vi "PTScanner.remove object.vi"(0 "i ref in":refnum<vi>, 2 "index":i32, 5 "error in (no error)":errorcluster) -> (14 "i ref out":refnum<vi>, 19 "error out":errorcluster)   [LabVIEW 2014, in "PTScanner.lvlib"]
uses:
  PTScanner.lvlib
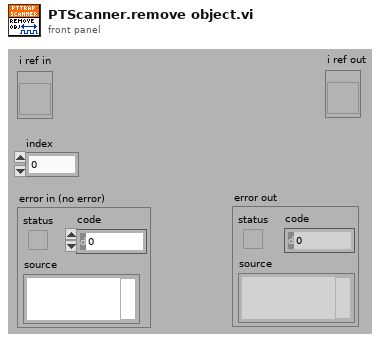
[diagram p1: front panel]
types:
  T1 = typedef "PTScanner.lvlib/PTScanner.i attribute.ctl" = cluster{"Object cmds":T2[], "Steps":cluster{"Finished":bool, "cmd setup":T3[]}[], "curStep":i32, "DIM IDs":cluster{"AllFinished":i32, "Finished":i32, "curStep":i32, "nofSteps":i32, "NomValues":i32[], "1D-Min":i32, "1D-Max":i32, "Dimensions":i32, "MaxDimensions":i32, "ScanedDeviceNames":i32[]}, "All Finished":bool, "DIMs in use":string[], "Running":bool, "Scan Delay":u32, "loop":bool, "Paused":bool, "Formed":bool}
  T2 = typedef "PTScanner.lvlib/PTScanner.obj parameters.ctl" = cluster{"object":string, "DIM address":string, "method":string, "data descriptor":string, "method parameters":cluster{"Name":string, "Descr":string, "Value":string, "Value?":bool}[], "Call Mode":enum16{"Simple DIM", "Synchronous"}, "actValue":dbl, "Centroid":dbl, "Minus Delta":dbl, "Plus Delta":dbl, "increment":dbl, "DIM Status":cluster{"no link":bool, "quality":i32, "Time Stamp":timestamp}, "range":dbl, "DIMChannelIndex":i32}
  T3 = typedef "PTScanner.lvlib/PTScanner.step obj parameters.ctl" = cluster{"obj index":i32, "nomValue":dbl, "fulfilled":bool}
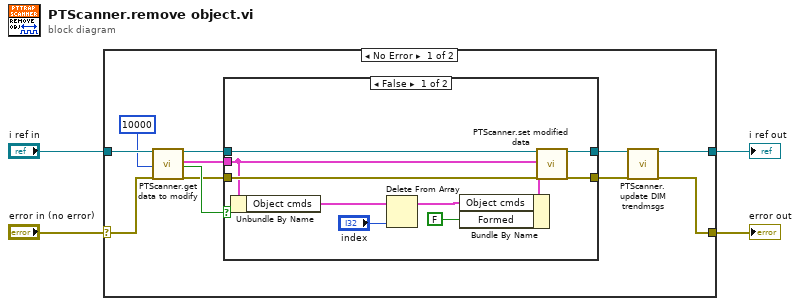
[diagram p0: block diagram]
diagram:
  n1 = case shown="No Error" "error in (no error)" {
    selector: "error in (no error)" -> [w10 w28]
    tunnel: "i ref in" -> [w11 w29]
    tunnel: [w7 w29] -> w2
    tunnel: [w5 w28] -> w1
    frame No Error {
      n2 = call "PTScanner.get data to modify.vi"("i ref in"=w11, "ms timeout (10000)"=10000, "error in (no error)"=w10) -> ("i ref out"=w14:refnum<vi>, "i attribute"=w12:T1, "timed out"=w15:bool, "error out"=w13:errorcluster)  [unwired: 13 in]
      n3 = case shown="False" w15 {
        tunnel: w14 -> [w25 w26]
        tunnel: w13 -> [w24 w27]
        tunnel: w12 -> [w23 _]
        tunnel: [w17 w27] -> w6
        tunnel: [w18 w26] -> w8
        frame False {
          n4 = Unbundle By Name(w23) -> ("Object cmds"=w21:T2[])
          n5 = Delete From Array(array=w21, index="index") -> (array with subset deleted=w20:T2[])  [unwired: 1 in, 1 out]
          n6 = Bundle By Name(cluster=w23, "Object cmds"=w20, "Formed"=FALSE) -> (w22:T1)
          n7 = call "PTScanner.set modified data.vi"("i ref in"=w25, "CLASS.i attribute"=w22, "error in (no error)"=w24) -> ("i ref out"=w18:refnum<vi>, "error out"=w17:errorcluster)  [unwired: 15 in]
        }
        frame True {
        }
      }
      n8 = call "PTScanner.update DIM trendmsgs.vi"("i ref in"=w8, "error in"=w6) -> ("i ref out"=w7:refnum<vi>, "error out"=w5:errorcluster)  [unwired: 16 in]
    }
    frame Error {
    }
  }
  "i ref out" <- w2
  "error out" <- w1
